vi "Process Counter Signals.vi"(9 "Values Received":dbl[](array[numeric]), 10 "Incoming Values In":T1, 11 "Frame Settings In":T2 {"Protection Configurations"."CRC Channels"."Data Type" items=["Signed", "Unsigned", "IEEE Float"]}) -> (1 "Values Received out":dbl[](array[numeric]), 2 "Incoming Values Out":T1, 3 "Frame Settings Out":T2 {"Protection Configurations"."CRC Channels"."Data Type" items=["Signed", "Unsigned", "IEEE Float"]})   [LabVIEW 2024, in "Protection and Counter Support Engine.lvlib"]
uses:
  Protection and Counter Support Engine.lvlib
  Types/RT Frame Settings.ctl
  Shared/Types/Exported Frame Type.ctl
  Types/RT Protection Configuration.ctl
  Shared/Types/Protection Type.ctl
  Shared/Types/XNET Signal Configuration.ctl
  Shared/Types/Exported Counter Settings.ctl
  Shared/Types/Exported Event Trigger Type.ctl
  Types/RT Frame Incoming Values.ctl
  Shared/Protection and Counter Support Shared.lvlib
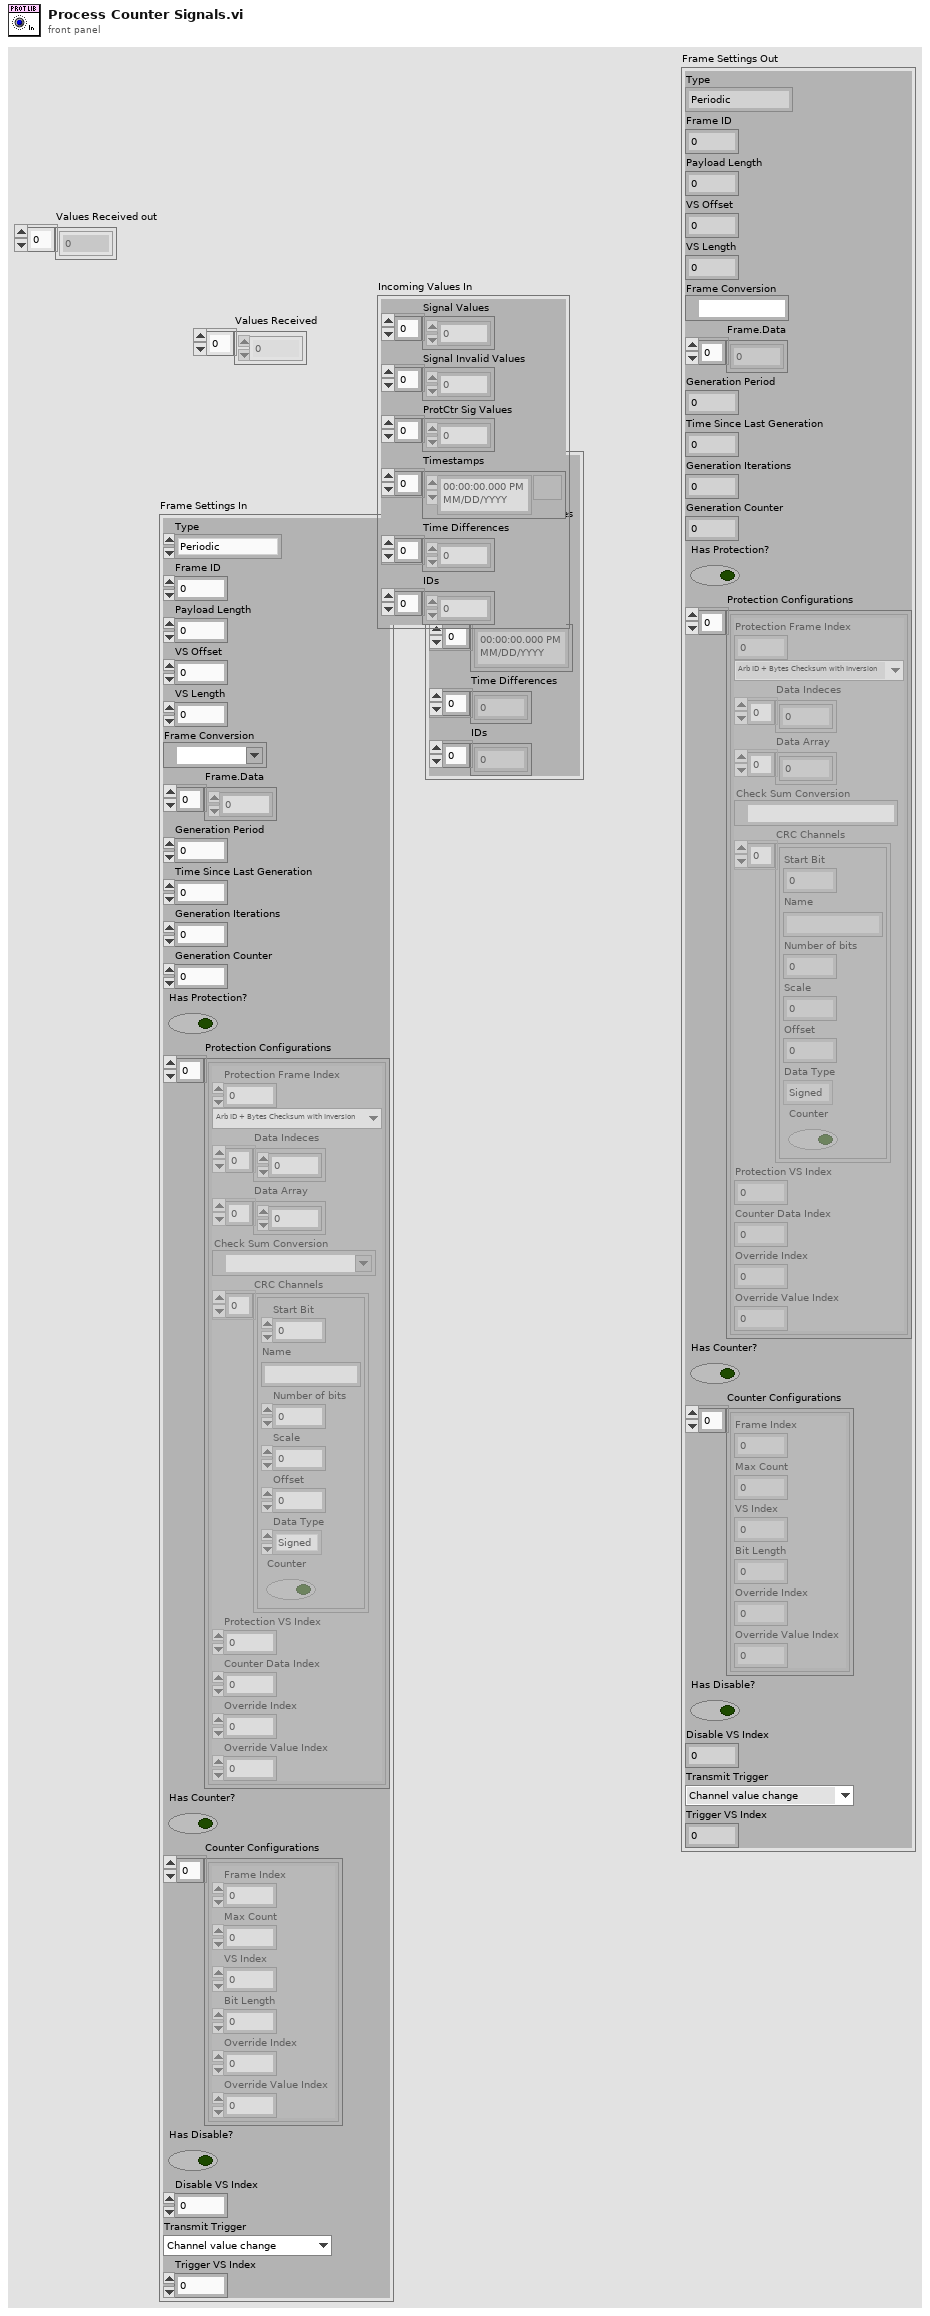
[diagram p1: front panel]
types:
  T1 = typedef "Protection and Counter Support Engine.lvlib/RT Frame Incoming Values.ctl" = cluster{"Signal Values":dbl[], "Signal Invalid Values":dbl[], "ProtCtr Sig Values":dbl[], "Timestamps":timestamp[], "Time Differences":dbl[], "IDs":u32[]}
  T2 = typedef "Protection and Counter Support Engine.lvlib/RT Frame Settings.ctl" = cluster{"Type":T3, "Frame ID":u32, "Payload Length":u32, "VS Offset":i32, "VS Length":i32, "Frame Conversion":refnum<k21>, "Frame.Data":dbl[], "Generation Period":u32, "Time Since Last Generation":u32, "Generation Iterations":u32, "Generation Counter":u32, "Has Protection?":bool, "Protection Configurations":T4[], "Has Counter?":bool, "Counter Configurations":T7[], "Has Disable?":bool, "Disable VS Index":i32, "Transmit Trigger":T8, "Trigger VS Index":i32}
  T3 = typedef "Protection and Counter Support Shared.lvlib/Exported Frame Type.ctl" = enum16{"Periodic", "Event", "Periodic/Event"}
  T4 = typedef "Protection and Counter Support Engine.lvlib/RT Protection Configuration.ctl" = cluster{"Protection Frame Index":i32, "Protection Type":T5, "Data Indeces":i32[], "Data Array":dbl[], "Check Sum Conversion":refnum<k21>, "CRC Channels":T6[], "Protection VS Index":i32, "Counter Data Index":i32, "Override Index":i32, "Override Value Index":i32}
  T5 = typedef "Protection and Counter Support Shared.lvlib/Protection Type.ctl" = enum16{"Arb ID + Bytes Checksum with Inversion", "Arb ID + Bytes CRC with Inversion", "Reversed Raw Signal Checksum with Inversion", "Concatenated Two's Compliment"}
  T6 = typedef "Protection and Counter Support Shared.lvlib/XNET Signal Configuration.ctl" = cluster{"Start Bit":i32, "Name":string, "Number of bits":i32, "Scale":dbl, "Offset":dbl, "Data Type":u32, "Counter":bool}
  T7 = typedef "Protection and Counter Support Shared.lvlib/Exported Counter Settings.ctl" = cluster{"Frame Index":i32, "Max Count":dbl, "VS Index":i32, "Bit Length":i64, "Override Index":i32, "Override Value Index":i32}
  T8 = typedef "Protection and Counter Support Shared.lvlib/Exported Event Trigger Type.ctl" = enum16{"Channel value change", "Trigger channel (not zero)", "Channel value change or trigger channel (not zero)", "Trigger channel (any value change)", "Channel value change or trigger channel (any value change)"}
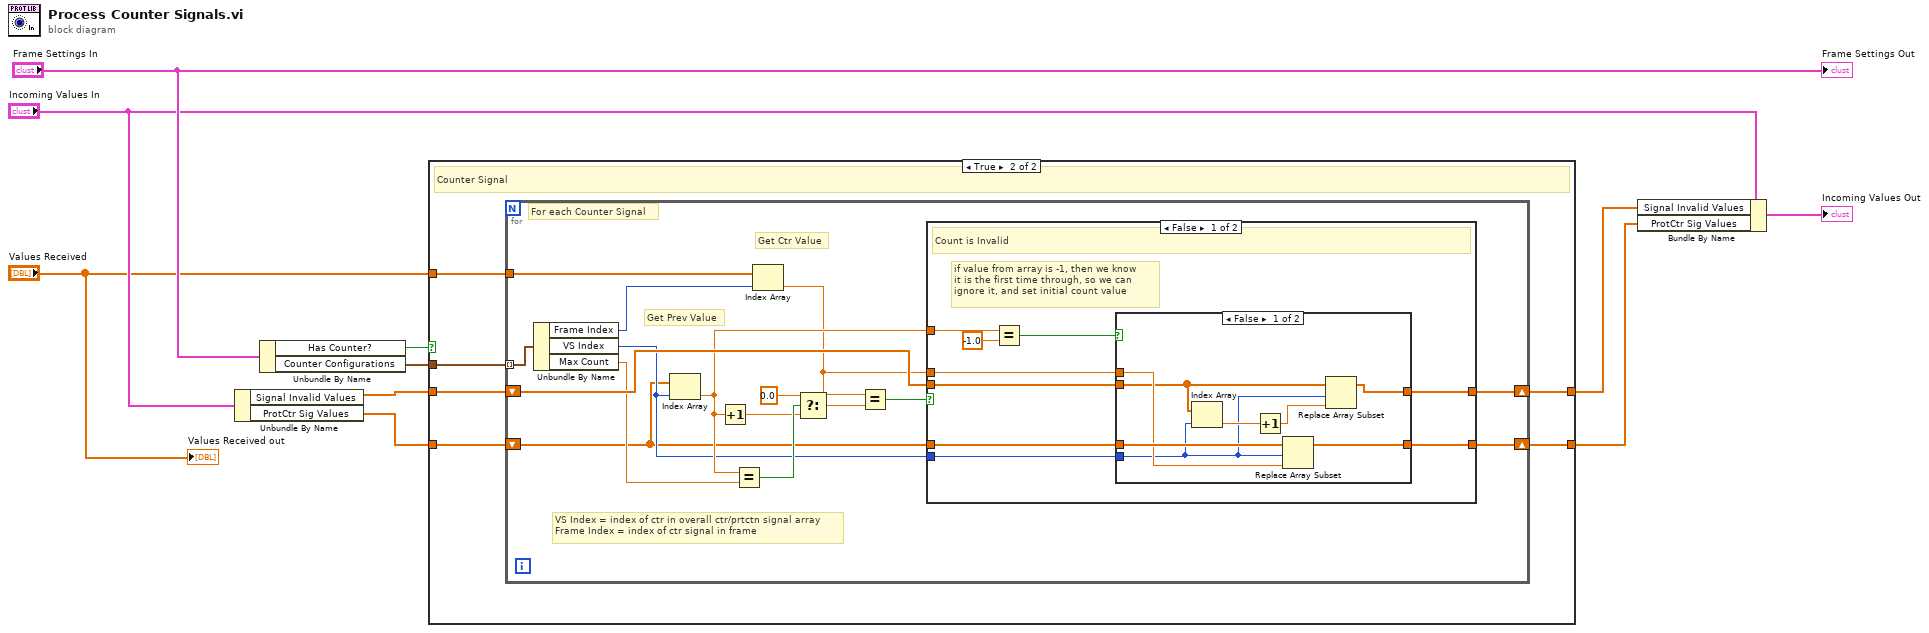
[diagram p0: block diagram]
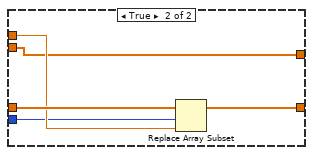
[diagram p3: hidden frame]
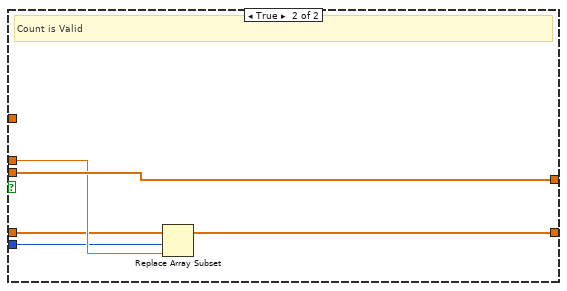
[diagram p4: hidden frame]
diagram:
  n1 = Unbundle By Name("Incoming Values In") -> ("Signal Invalid Values"=w3:dbl[], "ProtCtr Sig Values"=w2:dbl[])
  n2 = Unbundle By Name("Frame Settings In") -> ("Has Counter?"=w8:bool, "Counter Configurations"=w10:T7[])
  n3 = case shown="True" w8 {
    tunnel: "Values Received" -> [_ w15]
    tunnel: w3 -> [w12 w14]
    tunnel: w10 -> [_ w13]
    tunnel: [w12 w18] -> w5
    tunnel: w2 -> [w11 w16]
    tunnel: [w11 w17] -> w4
    frame False {
    }
    frame True {
      # "Counter Signal"
      n4 = for {
        tunnel: w15 -> [w22]
        tunnel: w13 -> [w25] mode=indexing
        shift-right: [w34] -> w18
        shift-left: w14 -> [w27]
        shift-right: [w33] -> w17
        shift-left: w16 -> [w19]
        # "Get Ctr Value"
        # "For each Counter Signal"
        # "VS Index = index of ctr in overall ctr/prtctn signal array\nFrame Index = index of ctr signal in frame"
        # "Get Prev Value"
        n5 = Unbundle By Name(w25) -> ("Frame Index"=w21:i32, "VS Index"=w23:i32, "Max Count"=w24:dbl)
        n6 = Index Array(array=w19, index=w23) -> (element=w26:dbl)
        n7 = Increment(x=w26) -> (x+1=w30:dbl)
        n8 = Equal?(x=w26, y=w24) -> (x = y?=w32:bool)
        n9 = Index Array(array=w22, index=w21) -> (element=w20:dbl)
        n10 = Select(t=0.0, s=w32, f=w30) -> (s? t:f=w29:dbl)
        n11 = Equal?(x=w20, y=w29) -> (x = y?=w28:bool)
        n12 = case shown="False" w28 {
          tunnel: w27 -> [w40 w61]
          tunnel: [w39 w61] -> w34
          tunnel: w20 -> [w42 w60]
          tunnel: [w41 w59] -> w33
          tunnel: w19 -> [w43 w58]
          tunnel: w26 -> [w38 _]
          tunnel: w23 -> [w35 w57]
          frame False {
            # "if value from array is -1, then we know \nit is the first time through, so we can\nignore it, and set initial count value"
            # "Count is Invalid"
            n13 = Equal?(x=w38, y=-1.0) -> (x = y?=w36:bool)
            n14 = case shown="False" w36 {
              tunnel: w43 -> [w51 w56]
              tunnel: w42 -> [w50 w55]
              tunnel: [w49 w54] -> w41
              tunnel: w40 -> [w48 w53]
              tunnel: [w45 w53] -> w39
              tunnel: w35 -> [w44 w52]
              frame False {
                n15 = Index Array(array=w48, index=w44) -> (element=w47:dbl)
                n16 = Increment(x=w47) -> (x+1=w46:dbl)
                n17 = Replace Array Subset(array=w51, new element=w50, index=w44) -> (w49:dbl[])
                n18 = Replace Array Subset(array=w48, new element=w46, index=w44) -> (w45:dbl[])
              }
              frame True {
                n19 = Replace Array Subset(array=w56, new element=w55, index=w52) -> (w54:dbl[])
              }
            }
          }
          frame True {
            # "Count is Valid"
            n20 = Replace Array Subset(array=w58, new element=w60, index=w57) -> (w59:dbl[])
          }
        }
      }
    }
  }
  n21 = Bundle By Name(cluster="Incoming Values In", "Signal Invalid Values"=w5, "ProtCtr Sig Values"=w4) -> (→"Incoming Values Out":T1)
  "Frame Settings Out" <- "Frame Settings In"
  "Values Received out" <- "Values Received"
